vi "readBoolean.vi"(8 "error in (no error)":errorcluster, 11 "IReadWriteControl in":refnum<class "IReadWriteControl.lvclass">) -> (0 "error out":errorcluster, 2 "Data":bool, 3 "IReadWriteControl out":refnum<class "IReadWriteControl.lvclass">)   [LabVIEW 2015, in "RTFPGA.lvlib" / "IReadWriteControl.lvclass"]
uses:
  IReadWriteControl.lvclass
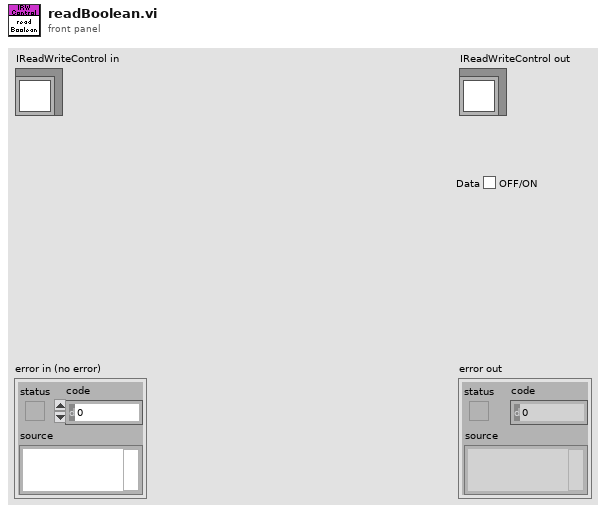
[diagram p1: front panel]
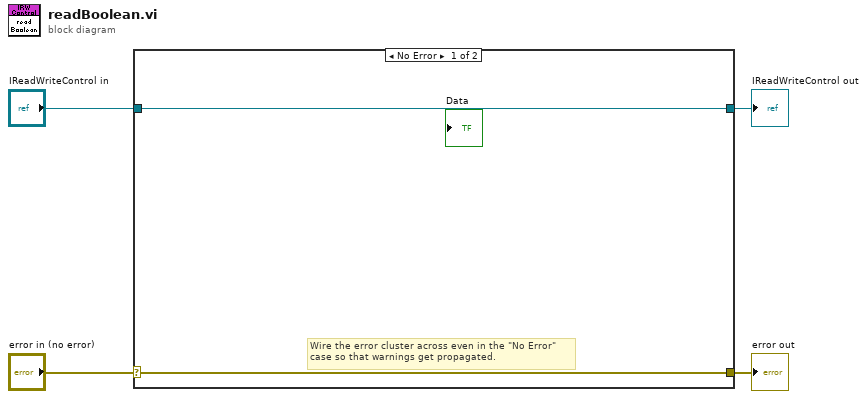
[diagram p0: block diagram]
diagram:
  n1 = case shown="No Error" "error in (no error)" {
    selector: "error in (no error)" -> [w5 w8]
    tunnel: [w5 w8] -> w3
    tunnel: [w6 w7] -> w1
    tunnel: "IReadWriteControl in" -> [w6 w7]
    frame No Error {
      # "Wire the error cluster across even in the \"No Error\"\ncase so that warnings get propagated."
    }
    frame Error {
    }
  }
  "error out" <- w3
  "IReadWriteControl out" <- w1
